vi "Error Dialog Main.vi"(8 "error in (no error)":errorcluster, 11 "Message in":string) -> (0 "error out":errorcluster)   [LabVIEW 2015, in "Error Dialog.lvclass"]
doc: "<b> </b> <b> </b>\n©2016 Q Software Innovations, LLC (QSI)\nwritten by Quentin Alldredge\nproduced in LabVIEW 2015\n\nsupport@qsoftwareinnovations.com\nwww.qsoftwareinnovations.com\n\nAll rights reserved.\n\nRedistribution and use in source and binary forms, with or without modification, are permitted provided that the following conditions are met:\n\n * Redistributions of source code must retain the above copyright notice, this list of conditions and the following disclaimer.\n * Redistributions in binary form must reproduce the above copyright notice, this list of conditions and the following disclaimer in the documentation and/or other materials provided with the distribution.\n * Neither the name of Q Software Innovations, LLC. nor the names of its contributors may be used to endorse or promote products derived from this software without specific prior written permission.\n\nTHIS SOFTWARE IS PROVIDED BY THE COPYRIGHT HOLDERS AND CONTRIBUTORS \"AS IS\" AND ANY EXPRESS OR IMPLIED WARRANTIES, INCLUDING, BUT NOT LIMITED TO, THE IMPLIED WARRANTIES OF MERCHANTABILITY AND FITNESS FOR A PARTICULAR PURPOSE ARE DISCLAIMED. IN NO EVENT SHALL THE COPYRIGHT OWNER OR CONTRIBUTORS BE LIABLE FOR ANY DIRECT, INDIRECT, INCIDENTAL, SPECIAL, EXEMPLARY, OR CONSEQUENTIAL DAMAGES (INCLUDING, BUT NOT LIMITED TO, PROCUREMENT OF SUBSTITUTE GOODS OR SERVICES; LOSS OF USE, DATA, OR PROFITS; OR BUSINESS INTERRUPTION) HOWEVER CAUSED AND ON ANY THEORY OF LIABILITY, WHETHER IN CONTRACT, STRICT LIABILITY, OR TORT (INCLUDING NEGLIGENCE OR OTHERWISE) ARISING IN ANY WAY OUT OF THE USE OF THIS SOFTWARE, EVEN IF ADVISED OF THE POSSIBILITY OF SUCH DAMAGE."
uses:
  Error Dialog.lvclass
  Dialog/Dialog.lvclass
panel:
  in  "OK":bool
  out "Message":string
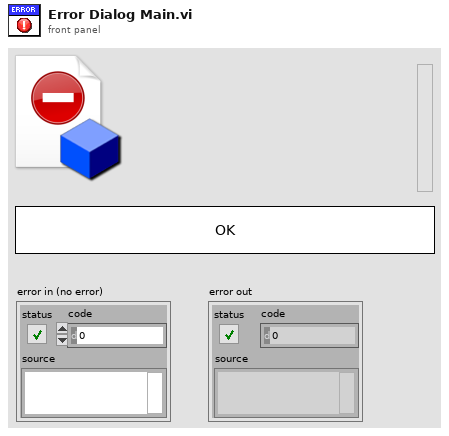
[diagram p1: front panel]
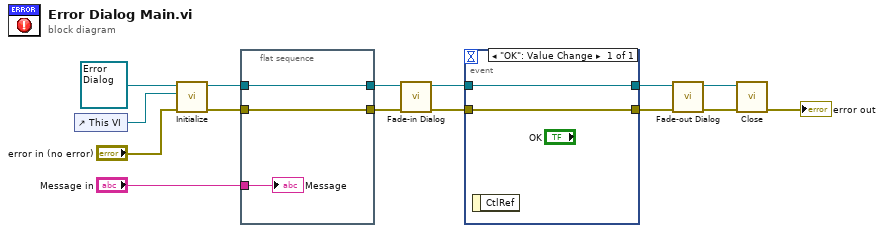
[diagram p0: block diagram]
diagram:
  n1 = control-ref of="This VI"() -> (w15:refnum<vi>)
  n2 = call-dynamic "Initialize.vi"("error in (no error)"="error in (no error)", "VI Refnum"=w15, "Error Dialog in"=refnum<class "Error Dialog.lvclass"> refnum ("ErrorDialog")) -> ("error out"=w10:errorcluster, "Error Dialog out"=w12:refnum<class "Error Dialog.lvclass">)  [unwired: 7 in]
  n3 = flat-sequence {
    tunnel: "Message in" -> [w18]
    tunnel: [w17] -> w13
    tunnel: w12 -> [w17]
    tunnel: [w16] -> w11
    tunnel: w10 -> [w16]
    frame #0 {
      "Message" <- w18
    }
  }
  n4 = call "Fade-in Dialog.vi"("error in (no error)"=w11, "Dialog in"=w13) -> ("error out"=w9:errorcluster, "Dialog out"=w8:refnum<class "Error Dialog.lvclass">)  [unwired: 8 in]
  n5 = event shown="[0] \"OK\": Value Change" {
    selector: _ -> [_]
    dyn-events: _ -> [_]
    timeout: _ -> [_]
    tunnel: w9 -> [w19]
    tunnel: w8 -> [w20]
    tunnel: [w20] -> w7
    tunnel: [w19] -> w6
    event "OK": Value Change {
      n6 = event-data() -> ()  [unwired: 1 in, 1 out]
    }
  }
  n7 = call "Fade-out Dialog.vi"("error in (no error)"=w6, "Dialog in"=w7) -> ("error out"=w4:errorcluster, "Dialog out"=w5:refnum<class "Error Dialog.lvclass">)  [unwired: 8 in]
  n8 = call-dynamic "Close.vi"("error in (no error)"=w4, "Dialog in"=w5) -> ("error out"=→"error out":errorcluster)  [unwired: 9 in]
